vi "Shutdown_Criteria_HGB2_rev01.vi"(8 "error in (no error)":errorcluster, 9 "Dummy Variable 2":dbl=100.0, 11 "Data Array":dbl[](array[numeric])=[27.384641856455705, 33.799845856644986, -57723.241032469305, 27.867724677726756, 16.018064048774477, 22.694692235265137, 16.554202451522293, 34.69000275563163, -57723.241032469305, -57723.241032469305, -57723.241032469305, -57723.241032469305, -57723.241032469305, -57723.241032469305, -57723.241032469305, -57723.241032469305, -0.03138978283403837, -0.2662265423540802, 508.87447056741576, 532.5490567913932, 514.3509121948407, 0.004466269370719865, 1.2172940638240613e-06, -0.0008776677125047275, 0.9108136314898729, 0.9830234628170729, 0.6065007708966732, 0.838603800162673, 0.9778656177222729, 0.781867504119873, 0.5755537003278732, 1.0500754490494728, 0.6993419826030731, 0.817972419783473, 444.7878360748291, 446.8509741127491, 440.6615599989891, 448.9141121506691, 440.6615599989891, 455.1035262644291, 432.4090078473091, 463.3560784161091, 459.2298023402691, 450.9772501885891]) -> (0 "error out":errorcluster, 3 "Boolean":bool)   [LabVIEW 2016]
panel:
  out "Superheat Maximum":bool
  out "Suction Pressure Limit":bool
  out "Superheat Minimum":bool
  out "Torque Limit":bool
  out "Discharge Pressure Limit":bool
  out "Discharge Temp Limit":bool
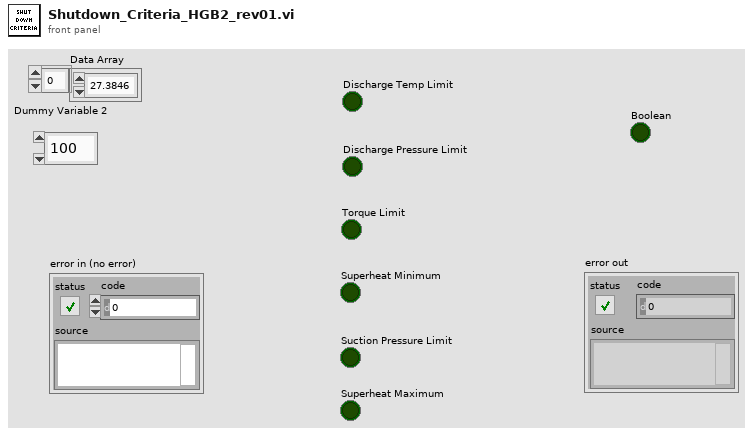
[diagram p1: front panel]
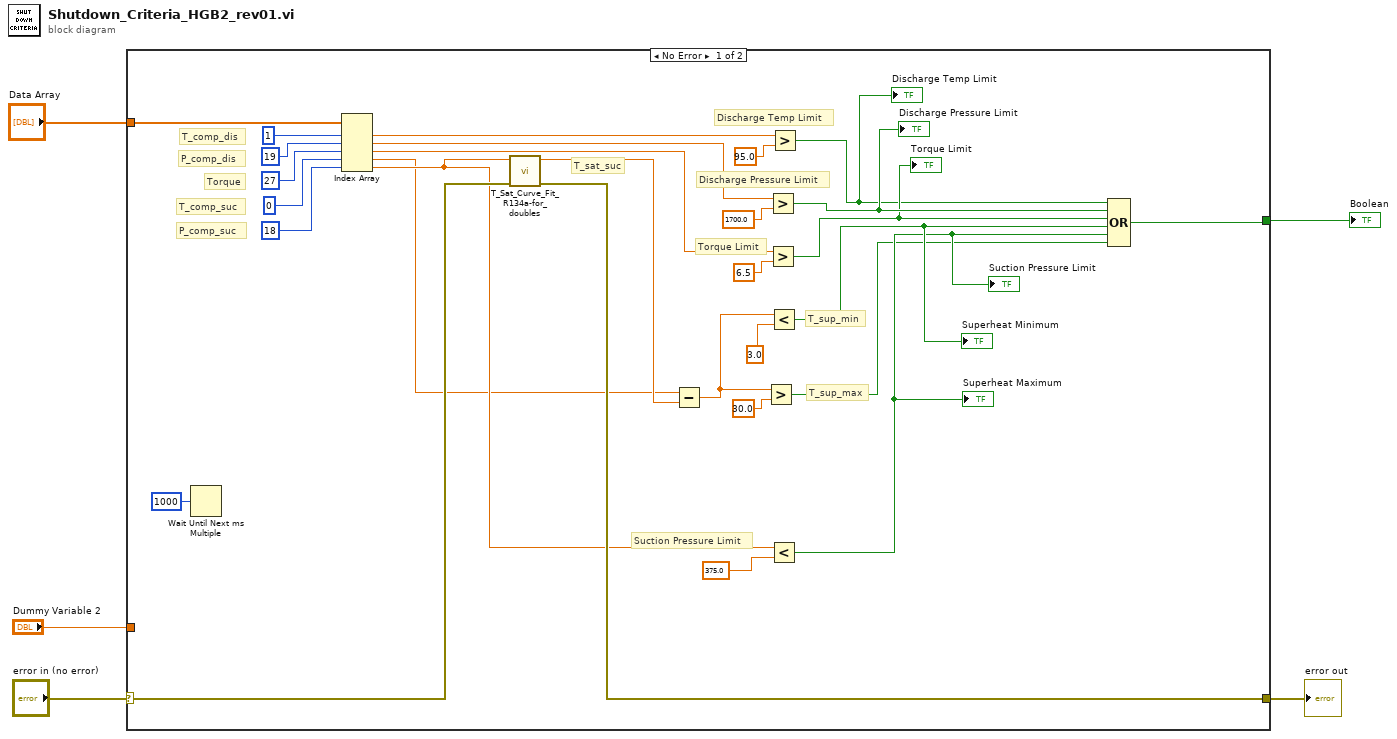
[diagram p0: block diagram]
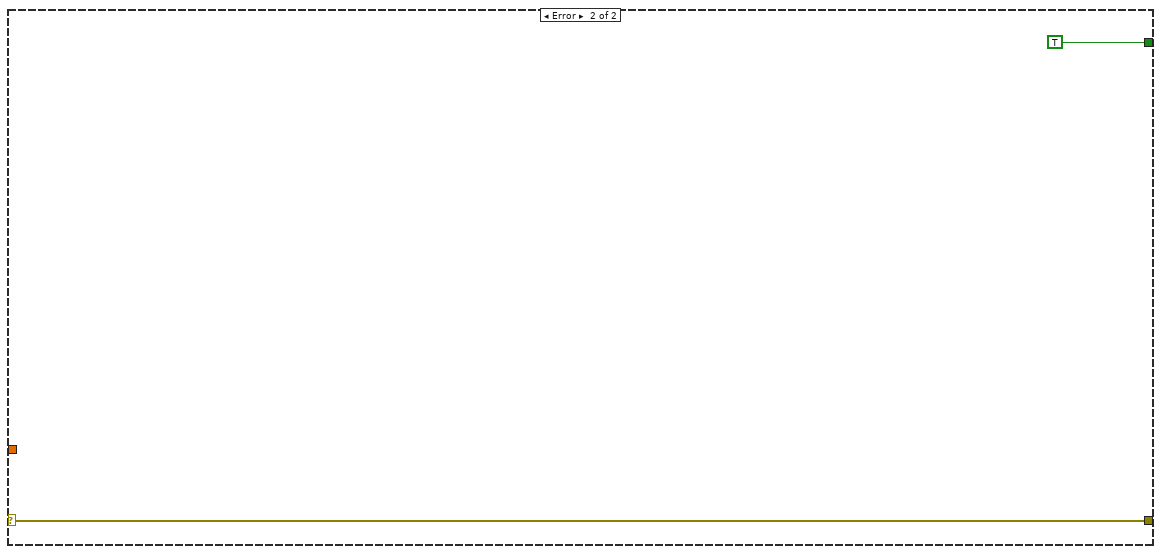
[diagram p2: hidden frame]
diagram:
  n1 = case shown="No Error" "error in (no error)" {
    selector: "error in (no error)" -> [w17 w36]
    tunnel: "Data Array" -> [w32 _]
    tunnel: [w16 w36] -> w3
    tunnel: "Dummy Variable 2" -> [_ _]
    tunnel: [w10 TRUE] -> w1
    frame No Error {
      # "T_sup_max"
      # "Suction Pressure Limit"
      # "Torque Limit"
      # "Discharge Pressure Limit"
      # "Discharge Temp Limit"
      # "T_sup_min"
      # "T_sat_suc"
      # "P_comp_suc"
      # "T_comp_suc"
      # "Torque"
      # "P_comp_dis"
      # "T_comp_dis"
      n2 = Wait Until Next ms Multiple(millisecond multiple=u32 1000) -> ()  [unwired: 1 out]
      n3 = Index Array(array=w32, index #1=1 ("index"), index #2=19 ("index"), index #3=27 ("index"), index #4=0 ("index"), index #5=18 ("index")) -> (element #1=w9:dbl, element #2=w26:dbl, element #3=w23:dbl, element #4=w13:dbl, element #5=w15:dbl)
      n4 = call "T_Sat_Curve_Fit_R134a-for_doubles.vi"("error in (no error)"=w17, "Numeric in"=w15) -> ("error out"=w16:errorcluster, "Numeric out"=w14:dbl)  [unwired: 8 in]
      n5 = Subtract(x=w13, y=w14) -> (x-y=w8:dbl)
      n6 = Greater?(x=w8, y=30.0) -> (0:w6:bool)
      n7 = Greater?(x=w26, y=1700.0) -> (0:w25:bool)
      "Discharge Pressure Limit" <- w25
      n8 = Greater?(x=w23, y=6.5) -> (0:w22:bool)
      "Torque Limit" <- w22
      n9 = Less?(x=w8, y=3.0) -> (x < y?=w19:bool)
      "Superheat Minimum" <- w19
      n10 = Less?(x=w15, y=375.0) -> (x < y?=w18:bool)
      "Suction Pressure Limit" <- w18
      "Superheat Maximum" <- w18
      n11 = Greater?(x=w9, y=95.0) -> (0:w11:bool)
      "Discharge Temp Limit" <- w11
      n12 = Compound Arithmetic op=OR(w11, w25, w22, w19, w18, w6) -> (w10:bool)
    }
    frame Error {
    }
  }
  "error out" <- w3
  "Boolean" <- w1
